vi "Handle Error.vi"(8 "error in (no error)":errorcluster, 11 "Function in":refnum<class "Function.lvclass">) -> (0 "error out":errorcluster, 2 "stop actor?":bool=TRUE, 3 "Function out":refnum<class "Function.lvclass">)   [LabVIEW 2016, in "Function Actor.lvlib" / "Function.lvclass"]
doc: "(<B>Filename</B>: Actor Framework.lvlib:Actor.lvclass:Handle Error.vi)\n\nDefines how the actor handles an error that occurred while processing a message.\n\nBy default, this method does nothing except stop the actor. This method also treats error code 43 (coming from <B>error in</B>) as a sign that the actor shut down normally. In this situation, the Handle Error method does not return the error on <B>error out</B>, meaning the actor's caller will not receive it. All other error codes will be returned on <B>error out</B>.\n\nA descendant class may override this method to change this behavior."
uses:
  <userlib>/Common Components/Function Actor/Function.lvclass
  C:/Program Files (x86)/National Instruments/LabVIEW 2016/vi.lib/ActorFramework/Actor/Actor.lvclass
  <vilib>/Utility/error.llb/DialogType.ctl
  <vilib>/ActorFramework/Actor/Actor.lvclass/Actor.ctl
  <vilib>/ActorFramework/Message Enqueuer/Message Enqueuer.lvclass/Message Enqueuer.ctl
  <userlib>/Common Components/Function Messages/Log in MsgList Msg/Log in MsgList Msg.lvclass/Log in MsgList Msg.ctl
  <vilib>/ActorFramework/Message Enqueuer/Init from Existing Queue.vi
  <vilib>/ActorFramework/Message Enqueuer/Enqueue.vi
  <userlib>/Common Components/Function Messages/Log in MsgList Msg/Log in MsgList Msg.lvclass
  C:/Program Files (x86)/National Instruments/LabVIEW 2016/vi.lib/ActorFramework/Message/Message.lvclass
  <vilib>/ActorFramework/Message Priority Queue/Priority Enqueue.vi
  <vilib>/ActorFramework/Message Enqueuer/Message Enqueuer.lvclass
  <userlib>/Common Components/Controller/Messages/Log Status/Log Status.lvclass
  <vilib>/ActorFramework/Actor/Actor.lvclass
  <userlib>/Common Components/Controller Messages/Request Stop Msg/Request Stop Msg.lvclass
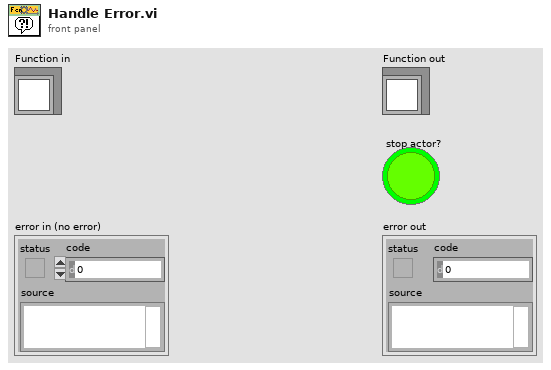
[diagram p1: front panel]
types:
  T1 = typedef "DialogType.ctl" = u16
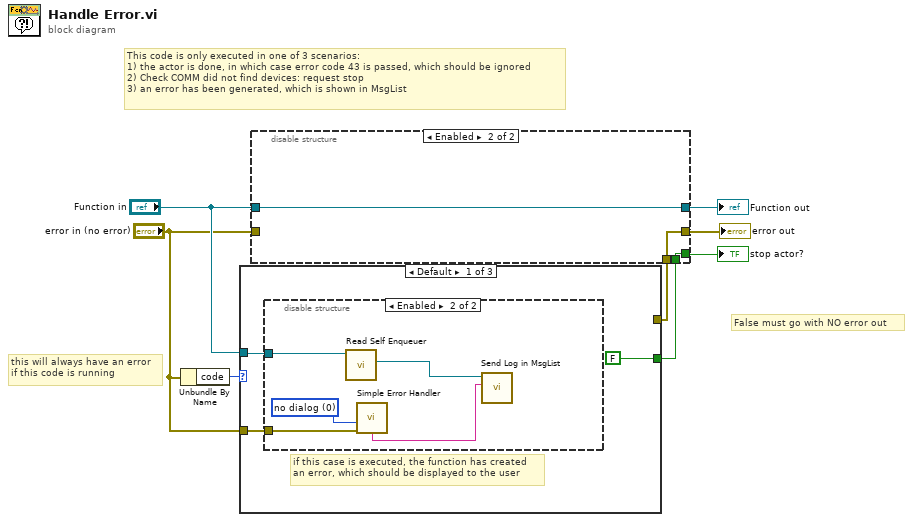
[diagram p0: block diagram]
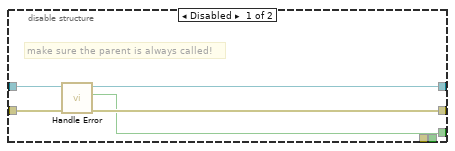
[diagram p2: hidden frame]
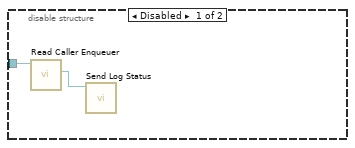
[diagram p3: hidden frame]
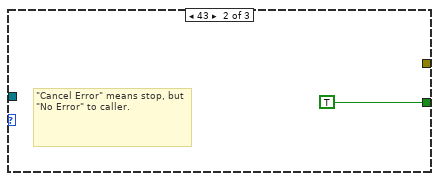
[diagram p4: hidden frame]
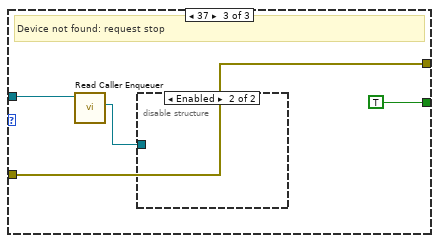
[diagram p5: hidden frame]
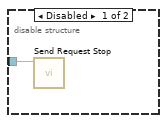
[diagram p6: hidden frame]
diagram:
  # "False must go with NO error out"
  # "this will always have an error\nif this code is running"
  # "This code is only executed in one of 3 scenarios:\n1) the actor is done, in which case error code 43 is passed, which should be ignored\n2) Check COMM did not find devices: request stop\n3) an error has been generated, which is shown in MsgList"
  n1 = Unbundle By Name("error in (no error)") -> ("code"=w4:i32)
  n2 = case shown="Default" w4 {
    tunnel: "Function in" -> [w11 _ w24]
    tunnel: [FALSE TRUE TRUE] -> w3
    tunnel: "error in (no error)" -> [w9 _ w21]
    tunnel: [_ _ w21] -> w1
    frame Default {
      # "if this case is executed, the function has created\nan error, which should be displayed to the user"
      n3 = disable-structure shown="Enabled" {
        disable-tunnel: w11 -> [w13 w18]
        disable-tunnel: w9 -> [_ w16]
        frame Disabled {
          n4 = call <vilib>:"Read Caller Enqueuer.vi"("Actor"=w13) -> ("Caller Enqueuer"=w14:refnum<class "Message Enqueuer.lvclass">)  [unwired: 10 in]
          n5 = call <userlib>:"Send Log Status.vi"("Message Enqueuer in"=w14) -> ("String"=w12:string)  [unwired: 8 in, 2 out]
        }
        frame Enabled {
          w17 = T1 0 items=["no dialog", "OK message", "continue or stop message", "OK message + warnings", "continue/stop + warnings"] ("type of dialog (OK msg:1)")
          n6 = call <vilib>:"Read Self Enqueuer.vi"("Actor"=w18) -> ("Self Enqueuer"=w19:refnum<class "Message Enqueuer.lvclass">)  [unwired: 10 in]
          n7 = call <vilib>:"Simple Error Handler.vi"("type of dialog (OK msg:1)"=w17, "error in (no error)"=w16) -> ("message"=w15:string)  [unwired: 3 in, 4 out]
          n8 = call <userlib>:"Send Log in MsgList.vi"("Msg"=w15, "Message Enqueuer"=w19) -> ()  [unwired: 8 in, 2 out]
        }
      }
    }
    frame 43 {
      # "\"Cancel Error\" means stop, but \"No Error\" to caller."
    }
    frame 37 {
      # "Device not found: request stop"
      n9 = call <vilib>:"Read Caller Enqueuer.vi"("Actor"=w24) -> ("Caller Enqueuer"=w23:refnum<class "Message Enqueuer.lvclass">)  [unwired: 10 in]
      n10 = disable-structure shown="Enabled" {
        disable-tunnel: w23 -> [w25 _]
        frame Disabled {
          n11 = call <userlib>:"Send Request Stop.vi"("Message Enqueuer"=w25) -> ()  [unwired: 9 in, 2 out]
        }
        frame Enabled {
        }
      }
    }
  }
  n12 = disable-structure shown="Enabled" {
    disable-tunnel: [w30 w31] -> w8
    disable-tunnel: [w29 w32] -> w7
    disable-tunnel: [w28 w33] -> w6
    disable-tunnel: "Function in" -> [w27 w33]
    disable-tunnel: "error in (no error)" -> [w26 _]
    disable-tunnel: w3 -> [_ w32]
    disable-tunnel: w1 -> [_ w31]
    frame Disabled {
      # "make sure the parent is always called!"
      n13 = call-parent "Handle Error.vi"("error in (no error)"=w26, "Actor in"=w27) -> ("error out"=w30:errorcluster, "stop actor?"=w29:bool, "Actor out"=w28:refnum<class "Function.lvclass">)  [unwired: 7 in]
    }
    frame Enabled {
    }
  }
  "Function out" <- w6
  "error out" <- w8
  "stop actor?" <- w7
